vi "Notify Response.vi"(8 "error in (no error)":errorcluster, 10 "Server Message":refnum<class "Server Message.lvclass">, 11 "OBS in":refnum<class "OBS.lvclass">) -> (0 "error out":errorcluster, 3 "OBS out":refnum<class "OBS.lvclass">)   [LabVIEW 2020, in "obs-websocket.lvlib" / "OBS.lvclass"]
uses:
  OBS.lvclass
  Server Message/Server Message.lvclass
  Response/Response.lvclass
  OBS.lvclass/OBS.ctl
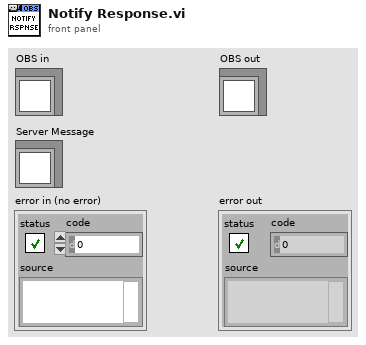
[diagram p1: front panel]
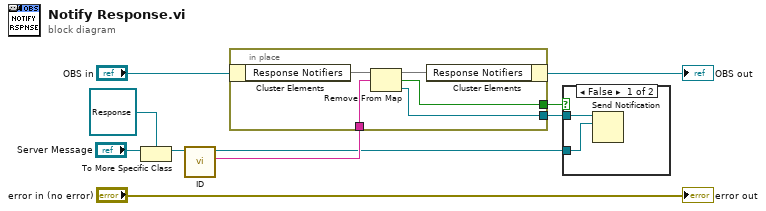
[diagram p0: block diagram]
diagram:
  n1 = To More Specific Class(target class=refnum<class "Response.lvclass"> refnum ("obs-websocket-lv.lvlib:Response.lvclass"), reference="Server Message") -> (specific class reference=w6:refnum<class "Response.lvclass">)  [unwired: 1 in, 1 out]
  n2 = call "ID.vi"("Response in"=w6) -> ("ID"=w5:string, "Response out"=w2:refnum<class "Response.lvclass">)  [unwired: 8 in, 1 out]
  n3 = in-place {
    in-place-border: w5 -> [w13]
    in-place-border: [w12] -> w3
    in-place-border: [w11] -> w4
    n4 = in-place-cluster #1("OBS in") -> ("Response Notifiers"=w15:map{string, refnum<notifier>})
    n5 = Remove From Map(10:w13, 11:w15) -> (1:w12:refnum<notifier>, 2:w11:bool, 3:w14:map{string, refnum<notifier>})
    n6 = in-place-cluster #1("Response Notifiers"=w14) -> (→"OBS out":refnum<class "OBS.lvclass">)
  }
  n7 = case shown="False" w4 {
    tunnel: w3 -> [w17 _]
    tunnel: w2 -> [w16 _]
    frame False {
      n8 = Send Notification(notification=w16, notifier=w17) -> ()  [unwired: 1 in, 2 out]
    }
    frame True {
      # "#ERROR?"
    }
  }
  "error out" <- "error in (no error)"
